vi "emi_ Loop error state monitor.vi"(5 "Loop ID in":u16, 9 "error in (no error)":errorcluster, 13 "Elevated priority":bool) -> (6 "Loop ID out":u16, 10 "error out":errorcluster)   [LabVIEW 2011]
doc: "Sends an E&S message when the error state in of this VI changes. \n\nDoes not remov ethe error"
uses:
  emi_Read System ID.vi
  Private/_emi_GFV System ID.vi
  <vilib>/Utility/error.llb/Clear Errors.vi
  S&E reporting/Private/_emi_S&E Q Generator.vi
panel:
  # "Always uses Sub ID 0."
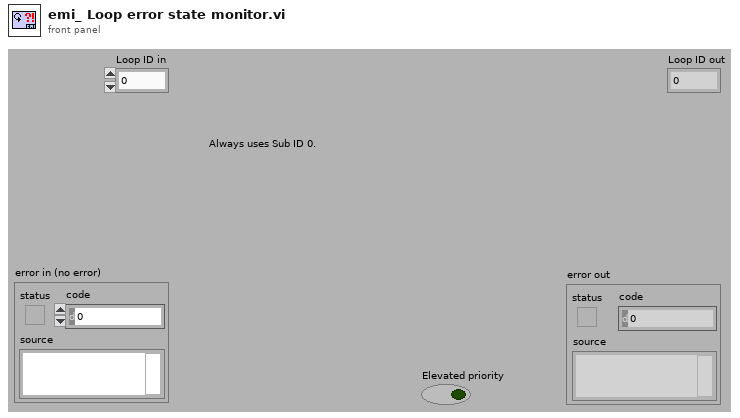
[diagram p1: front panel]
types:
  T1 = cluster{"error in (no error)":errorcluster, "Elevated priority":bool}
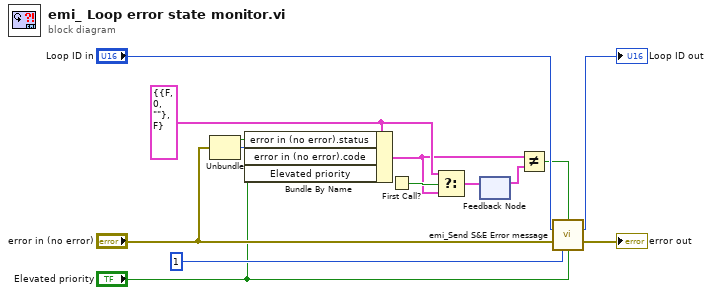
[diagram p0: block diagram]
diagram:
  w3 = T1 {"error in (no error)"={"status"=FALSE, "code"=0, "source"=""}, "Elevated priority"=FALSE}
  n1 = Unbundle("error in (no error)") -> ("status"=w6:bool, "code"=w5:i32)  [unwired: 1 out]
  n2 = Bundle By Name(cluster=w3, "error in (no error).status"=w6, "error in (no error).code"=w5, "Elevated priority"="Elevated priority") -> (w2:T1)
  n3 = First Call?() -> (First Call?: T/F=w4:bool)
  n4 = Select(t=w3, s=w4, f=w2) -> (s? t:f=w1:T1)
  n5 = feedback-in #1(w1) -> ()
  n6 = feedback #1() -> (w11:T1)  [unwired: 1 in]
  n7 = Not Equal?(x=w2, y=w11) -> (x != y?=w10:bool)
  n8 = call "emi_Send S&E Error message.vi"("Send(T)"=w10, "Loop ID in(No Loop)"="Loop ID in", "error in (no error)"="error in (no error)", "Var Index"=u16 1 ("Loc Sub ID"), "Elevated priority"="Elevated priority") -> ("Loop ID out"=→"Loop ID out":u16, "error out"=→"error out":errorcluster)  [unwired: 9 in]
